vi "Configure Measurements (Ballast).vi"(8 "error in (no error)":errorcluster, 10 "Ballast Measurements":i32[](listbox)=[0, 1, 2, 5, 6], 11 "VISA resource name":refnum<visa-resource-name>) -> (0 "error out":errorcluster, 3 "VISA resource name out":refnum<visa-resource-name>)   [LabVIEW 2015, in "Voltech PM1000+.lvlib"]
doc: "Configures the measurement itmes. This vi can only be used when PM1000+ is set to Ballast mode by using \"Configure Mode\" vi."
uses:
  <instrlib>/Voltech PM1000+/Voltech PM1000+.lvlib
panel:
  # "Notice:  \nHold \"Ctrl\" key and click the \nmeasurements to select \nmultiple items."
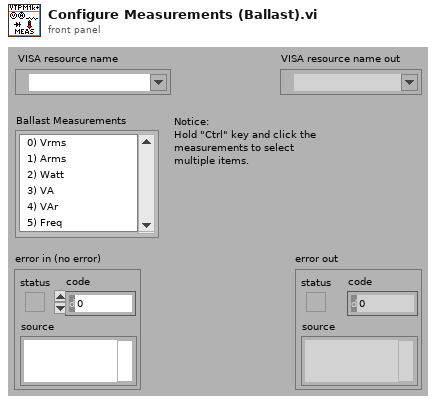
[diagram p1: front panel]
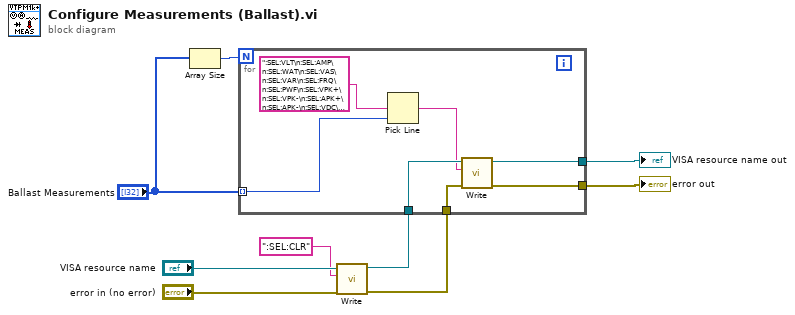
[diagram p0: block diagram]
diagram:
  n1 = Array Size(array="Ballast Measurements") -> (size(s)=w9:i32)
  n2 = call <instrlib>:"Write.vi"("error in (no error)"="error in (no error)", "Write Buffer"=":SEL:CLR" ("multi-line string"), "VISA resource name"="VISA resource name") -> ("error out"=w4:errorcluster, "VISA resource name out"=w5:refnum<visa-resource-name>)  [unwired: 7 in]
  n3 = for {
    N: w9 -> [_]
    tunnel: "Ballast Measurements" -> [w15] mode=indexing
    tunnel: w5 -> [w14]
    tunnel: w4 -> [w13]
    tunnel: [w12] -> w2
    tunnel: [w11] -> w1
    n4 = Pick Line(multi-line string=":SEL:VLT\n:SEL:AMP\n:SEL:WAT\n:SEL:VAS\n:SEL:VAR\n:SEL:FRQ\n:SEL:PWF\n:SEL:VPK+\n:SEL:VPK-\n:SEL:APK+\n:SEL:APK-\n:SEL:VDC\n:SEL:ADC\n:SEL:VCF\n:SEL:ACF\n:SEL:VDF\n:SEL:ADF\n:SEL:VHM\n:SEL:AHM\n:SEL:VRNG\n:SEL:ARNG", line index=w15) -> (output string=w10:string)  [unwired: 1 in]
    n5 = call <instrlib>:"Write.vi"("error in (no error)"=w13, "Write Buffer"=w10, "VISA resource name"=w14) -> ("error out"=w11:errorcluster, "VISA resource name out"=w12:refnum<visa-resource-name>)  [unwired: 7 in]
  }
  "error out" <- w1
  "VISA resource name out" <- w2
